vi "FindCurrentLevel.vi"(9 "value":dbl, 10 "latched severity":i32, 11 "rule":T1) -> (2 "severity out":i32)   [LabVIEW 2017, in "TrendAlarm.lvlib"]
uses:
  <vilib>/addons/InsightCM/Devices/Shared/Common/TrendAlarm/TrendAlarm.lvlib
  <vilib>/addons/InsightCM/MessageBus/Base/controls/TrendAlarmRule.ctl
  <vilib>/addons/InsightCM/MessageBus/Base/controls/TrendAlarmLevel.ctl
  <vilib>/addons/InsightCM/MessageBus/Base/controls/AlarmAction.ctl
  <vilib>/addons/InsightCM/MessageBus/Base/controls/KeyValuePair.ctl
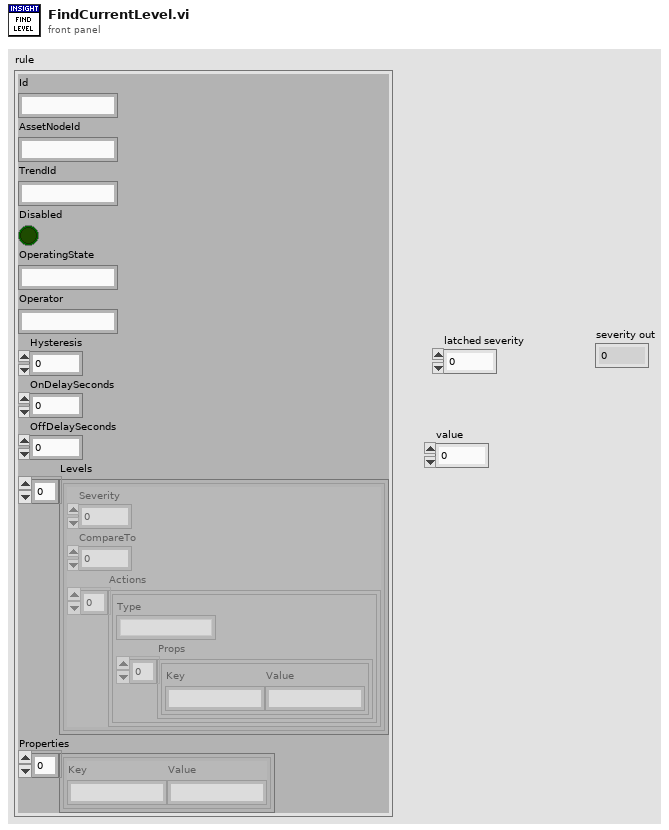
[diagram p1: front panel]
types:
  T1 = typedef "TrendAlarmRule.ctl" = cluster{"Id":string, "AssetNodeId":string, "TrendId":string, "Disabled":bool, "OperatingState":string, "Operator":string, "Hysteresis":dbl, "OnDelaySeconds":dbl, "OffDelaySeconds":dbl, "Levels":T2[], "Properties":T4[]}
  T2 = typedef "TrendAlarmLevel.ctl" = cluster{"Severity":i32, "CompareTo":dbl, "Actions":T3[]}
  T3 = typedef "AlarmAction.ctl" = cluster{"Type":string, "Props":T4[]}
  T4 = typedef "KeyValuePair.ctl" = cluster{"Key":string, "Value":string}
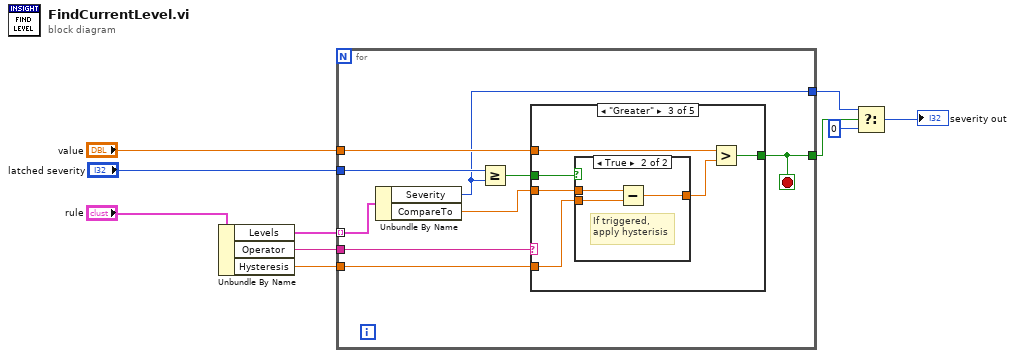
[diagram p0: block diagram]
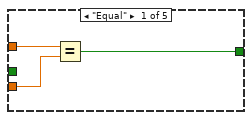
[diagram p2: hidden frame]
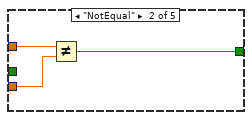
[diagram p3: hidden frame]
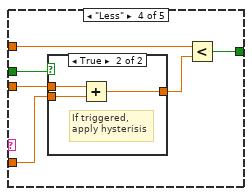
[diagram p5: hidden frame]
diagram:
  n1 = Unbundle By Name("rule") -> ("Levels"=w10:T2[], "Operator"=w7:string, "Hysteresis"=w8:dbl)
  n2 = for {
    tunnel: w10 -> [w12] mode=indexing
    tunnel: "value" -> [w19]
    tunnel: w8 -> [w17]
    tunnel: "latched severity" -> [w16]
    tunnel: w7 -> [w14]
    tunnel: [w13] -> w5
    tunnel: [w11] -> w4
    stop <- w13 stop-if-true
    n3 = Unbundle By Name(w12) -> ("Severity"=w11:i32, "CompareTo"=w18:dbl)
    n4 = Greater Or Equal?(x=w16, y=w11) -> (x >= y?=w15:bool)
    n5 = case shown="\"Greater\"" w14 {
      tunnel: w18 -> [w22 w25 w29 w40 _]
      tunnel: [w21 w24 w31 w41 _] -> w13
      tunnel: w19 -> [w20 w23 w27 w37 _]
      tunnel: w17 -> [_ _ w30 w39 _]
      tunnel: w15 -> [_ _ w26 w36 _]
      frame "Equal" {
        n6 = Equal?(x=w20, y=w22) -> (x = y?=w21:bool)
      }
      frame "NotEqual" {
        n7 = Not Equal?(x=w23, y=w25) -> (x != y?=w24:bool)
      }
      frame "Greater" {
        n8 = case shown="True" w26 {
          tunnel: w30 -> [_ w35]
          tunnel: w29 -> [w32 w34]
          tunnel: [w32 w33] -> w28
          frame False {
          }
          frame True {
            # "If triggered,\napply hysterisis"
            n9 = Subtract(x=w34, y=w35) -> (x-y=w33:dbl)
          }
        }
        n10 = Greater?(x=w27, y=w28) -> (0:w31:bool)
      }
      frame "Less" {
        n11 = case shown="True" w36 {
          tunnel: w40 -> [w42 w45]
          tunnel: w39 -> [_ w44]
          tunnel: [w42 w43] -> w38
          frame False {
          }
          frame True {
            # "If triggered,\napply hysterisis"
            n12 = Add(x=w45, y=w44) -> (x+y=w43:dbl)
          }
        }
        n13 = Less?(x=w37, y=w38) -> (x < y?=w41:bool)
      }
      frame Default {
      }
    }
  }
  n14 = Select(t=w4, s=w5, f=0) -> (s? t:f=→"severity out":i32)
